vi "Write Frame Data Recorder.vi"(8 "error in (no error)":errorcluster, 9 "Append":bool, 10 "Probe Position":T1, 11 "Frame Grabber Data In in":T5={"Camera Session"="", "Frame"=refnum, "AVI Refnum"=refnum, "Codecs"=[], "Frame number"=0, "Tracking File Refnum"=refnum, "Tick Count"=0, "Probe Object"=refnum, "Playback Probe Data"=[], "Rigid Body"={"Position"={"x (mm)"=0.0, "y (mm)"=0.0, "z (mm)"=0.0}, "Orientation"={"Pitch (rad)"=0.0, "Yaw (rad)"=0.0, "Roll (rad)"=0.0}, "Quaternion"={"qx"=0.0, "qy"=0.0, "qz"=0.0, "qw"=0.0}, "Tracked?"=FALSE}, "Total no frames playback"=0, "Video FPS"=0.0, "Camera connected?"=FALSE, "Scene"=refnum, "Cropped Frame"=refnum, "Tracker FPS"=0.0, "Crop ROI"=[], "Presentation Values"=[], "Elapsed time (ms)"=0, "Camera frames playback"=0, "Refnums"={"Live Refnum"=refnum, "Record Refnum"=refnum, "Playback Refnum"=refnum, "Frame Slider Refnum"=refnum, "Pause Refnum"=refnum, "Home Refnum"=refnum, "Set Crop Refnum"=refnum, "Clear Crop Refnum"=refnum, "stop refnum"=refnum, "Playback Rate Refnum"=refnum, "Presentation Refnum"=refnum, "Crop Time Frame Slider Refnum"=refnum, "Cancel Save Refnum"=refnum, "Reverse Playback Refnum"=refnum, "Recording Settings Refnum"=refnum, "Continuous Playback Refnum"=refnum, "Camera Frame Refnum"=refnum, "Annotation Refnum"=refnum, "Export All Refnum"=refnum, "Export List Refnum"=refnum, "Fill List Refnum"=refnum, "Save Crop Refnum"=refnum, "Skip Forward Refnum"=refnum, "Skip Backward Refnum"=refnum, "Single Annotation Refnum"=refnum, "Load Refnum"=refnum, "Set Start Refnum"=refnum, "Set End Refnum"=refnum, "Add to List Refnum"=refnum, "List of Annotations Refnum"=refnum}, "Dimensions"={"Probe Dimensions"={"Probe Width"=0.0, "Probe Depth"=1.0, "Probe Height"=0.0}, "Room Dimensions"={"Room Width"=0.0, "Room Depth"=0.0, "Room Height"=0.0}}, "Playback Data As Strings"=[], "Cropped Tracking File Refnum"=refnum, "Cropped AVI Refnum"=refnum, "Header"=[], "Total euclidian distance"=0.0, "Annotation File Path"=path "", "Playback File Path"=path "", "Size per frame"=0.0, "Ground Truth File Refnum"=refnum, "Annotation Array"=[], "Annotation TIFFs Folder"=path ""}) -> (0 "error out":errorcluster, 1 "Time elapsed (s)":dbl, 2 "Image":T4, 3 "Frame Grabber Data out":T5={"Camera Session"="", "Frame"=refnum, "AVI Refnum"=refnum, "Codecs"=[], "Frame number"=0, "Tracking File Refnum"=refnum, "Tick Count"=0, "Probe Object"=refnum, "Playback Probe Data"=[], "Rigid Body"={"Position"={"x (mm)"=0.0, "y (mm)"=0.0, "z (mm)"=0.0}, "Orientation"={"Pitch (rad)"=0.0, "Yaw (rad)"=0.0, "Roll (rad)"=0.0}, "Quaternion"={"qx"=0.0, "qy"=0.0, "qz"=0.0, "qw"=0.0}, "Tracked?"=FALSE}, "Total no frames playback"=0, "Video FPS"=0.0, "Camera connected?"=FALSE, "Scene"=refnum, "Cropped Frame"=refnum, "Tracker FPS"=0.0, "Crop ROI"=[], "Presentation Values"=[], "Elapsed time (ms)"=0, "Camera frames playback"=0, "Refnums"={"Live Refnum"=refnum, "Record Refnum"=refnum, "Playback Refnum"=refnum, "Frame Slider Refnum"=refnum, "Pause Refnum"=refnum, "Home Refnum"=refnum, "Set Crop Refnum"=refnum, "Clear Crop Refnum"=refnum, "stop refnum"=refnum, "Playback Rate Refnum"=refnum, "Presentation Refnum"=refnum, "Crop Time Frame Slider Refnum"=refnum, "Cancel Save Refnum"=refnum, "Reverse Playback Refnum"=refnum, "Recording Settings Refnum"=refnum, "Continuous Playback Refnum"=refnum, "Camera Frame Refnum"=refnum, "Annotation Refnum"=refnum, "Export All Refnum"=refnum, "Export List Refnum"=refnum, "Fill List Refnum"=refnum, "Save Crop Refnum"=refnum, "Skip Forward Refnum"=refnum, "Skip Backward Refnum"=refnum, "Single Annotation Refnum"=refnum, "Load Refnum"=refnum, "Set Start Refnum"=refnum, "Set End Refnum"=refnum, "Add to List Refnum"=refnum, "List of Annotations Refnum"=refnum}, "Dimensions"={"Probe Dimensions"={"Probe Width"=0.0, "Probe Depth"=1.0, "Probe Height"=0.0}, "Room Dimensions"={"Room Width"=0.0, "Room Depth"=0.0, "Room Height"=0.0}}, "Playback Data As Strings"=[], "Cropped Tracking File Refnum"=refnum, "Cropped AVI Refnum"=refnum, "Header"=[], "Total euclidian distance"=0.0, "Annotation File Path"=path "", "Playback File Path"=path "", "Size per frame"=0.0, "Ground Truth File Refnum"=refnum, "Annotation Array"=[], "Annotation TIFFs Folder"=path ""}, 4 "File Size (MB)":dbl, 5 "Greater than 2 GB?":bool)   [LabVIEW 2017]
uses:
  Controls/Frame Grabber Data.ctl
  <vilib>/userdefined/High Color/IMAQdx.ctl
  <vilib>/vision/Image Controls.llb/IMAQ Image.ctl
  <vilib>/vision/Avi.llb/IMAQ AVI2 Refnum.ctl
  Controls/Rigid Body Info.ctl
  Controls/Position.ctl
  Controls/Orientation.ctl
  Controls/Refnums.ctl
  Controls/Recording Settings.ctl
  Controls/Operator Settings.ctl
  Controls/Operator.ctl
  Controls/Patient Settings.ctl
  Controls/Dimensions.ctl
  Controls/Room Dimensions.ctl
panel:
  out "Camera frame number":dbl
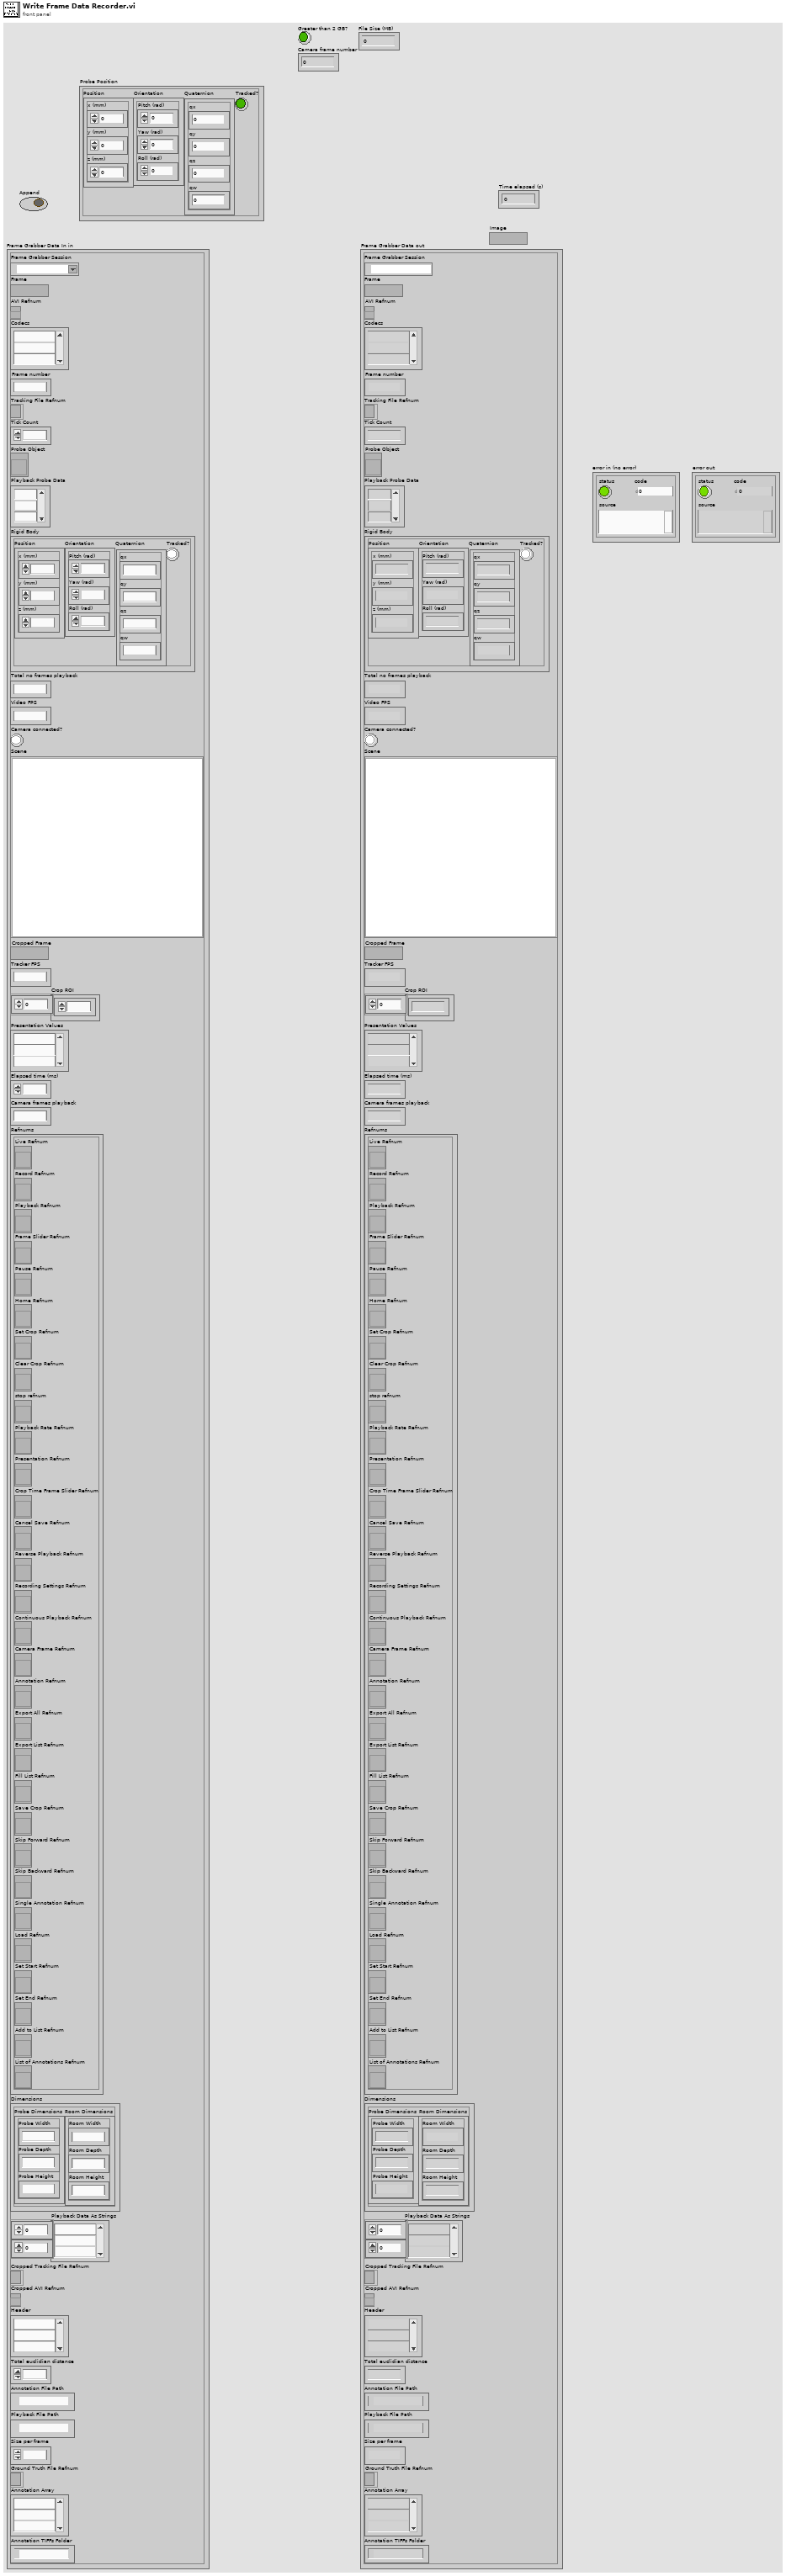
[diagram p1: front panel]
types:
  T1 = typedef "Rigid Body Info.ctl" = cluster{"Position":T2, "Orientation":T3, "Quaternion":cluster{"qx":sgl, "qy":sgl, "qz":sgl, "qw":sgl}, "Tracked?":bool}
  T2 = typedef "Position.ctl" = cluster{"x (mm)":sgl, "y (mm)":sgl, "z (mm)":sgl}
  T3 = typedef "Orientation.ctl" = cluster{"Pitch (rad)":sgl, "Yaw (rad)":sgl, "Roll (rad)":sgl}
  T4 = typedef "IMAQ Image.ctl" = refnum<image>
  T5 = typedef "Frame Grabber Data.ctl" = cluster{"Camera Session":T6, "Frame":T4, "AVI Refnum":T7, "Codecs":string[], "Frame number":u32, "Tracking File Refnum":refnum<file>, "Tick Count":u32, "Probe Object":refnum<vi>, "Playback Probe Data":dbl[][], "Rigid Body":T1, "Total no frames playback":i32, "Video FPS":dbl, "Camera connected?":bool, "Scene":refnum<vi>, "Cropped Frame":T4, "Tracker FPS":dbl, "Crop ROI":i32[], "Presentation Values":string[], "Elapsed time (ms)":u32, "Camera frames playback":u32, "Refnums":T8, "Dimensions":T9, "Playback Data As Strings":string[][], "Cropped Tracking File Refnum":refnum<file>, "Cropped AVI Refnum":T7, "Header":string[], "Total euclidian distance":dbl, "Annotation File Path":path, "Playback File Path":path, "Size per frame":dbl, "Ground Truth File Refnum":refnum<file>, "Annotation Array":string[], "Annotation TIFFs Folder":path}
  T6 = typedef "IMAQdx.ctl" = refnum<k21>
  T7 = typedef "IMAQ AVI2 Refnum.ctl" = refnum<k20>
  T8 = typedef "Refnums.ctl" = cluster{"Live Refnum":refnum<vi>, "Record Refnum":refnum<vi>, "Playback Refnum":refnum<vi>, "Frame Slider Refnum":refnum<vi>, "Pause Refnum":refnum<vi>, "Home Refnum":refnum<vi>, "Set Crop Refnum":refnum<vi>, "Clear Crop Refnum":refnum<vi>, "stop refnum":refnum<vi>, "Playback Rate Refnum":refnum<vi>, "Presentation Refnum":refnum<vi>, "Crop Time Frame Slider Refnum":refnum<vi>, "Cancel Save Refnum":refnum<vi>, "Reverse Playback Refnum":refnum<vi>, "Recording Settings Refnum":refnum<vi>, "Continuous Playback Refnum":refnum<vi>, "Camera Frame Refnum":refnum<vi>, "Annotation Refnum":refnum<vi>, "Export All Refnum":refnum<vi>, "Export List Refnum":refnum<vi>, "Fill List Refnum":refnum<vi>, "Save Crop Refnum":refnum<vi>, "Skip Forward Refnum":refnum<vi>, "Skip Backward Refnum":refnum<vi>, "Single Annotation Refnum":refnum<vi>, "Load Refnum":refnum<vi>, "Set Start Refnum":refnum<vi>, "Set End Refnum":refnum<vi>, "Add to List Refnum":refnum<vi>, "List of Annotations Refnum":refnum<vi>}
  T9 = typedef "Dimensions.ctl" = cluster{"Probe Dimensions":cluster{"Probe Width":sgl, "Probe Depth":sgl, "Probe Height":sgl}, "Room Dimensions":T10}
  T10 = typedef "Room Dimensions.ctl" = cluster{"Room Width":dbl, "Room Depth":dbl, "Room Height":dbl}
  T11 = typedef "Recording Settings.ctl" = cluster{"Folder to Save Recordings":path, "Video FPS":u32, "Codec":u16, "Tracker FPS":u32, "Operator ID":T12, "Patient ID/Gestation":T14}
  T12 = typedef "Operator Settings.ctl" = cluster{"Operator ID":u32, "Expertise":T13}
  T13 = typedef "Operator.ctl" = u16
  T14 = typedef "Patient Settings.ctl" = cluster{"ID":u32, "Gestation":string}
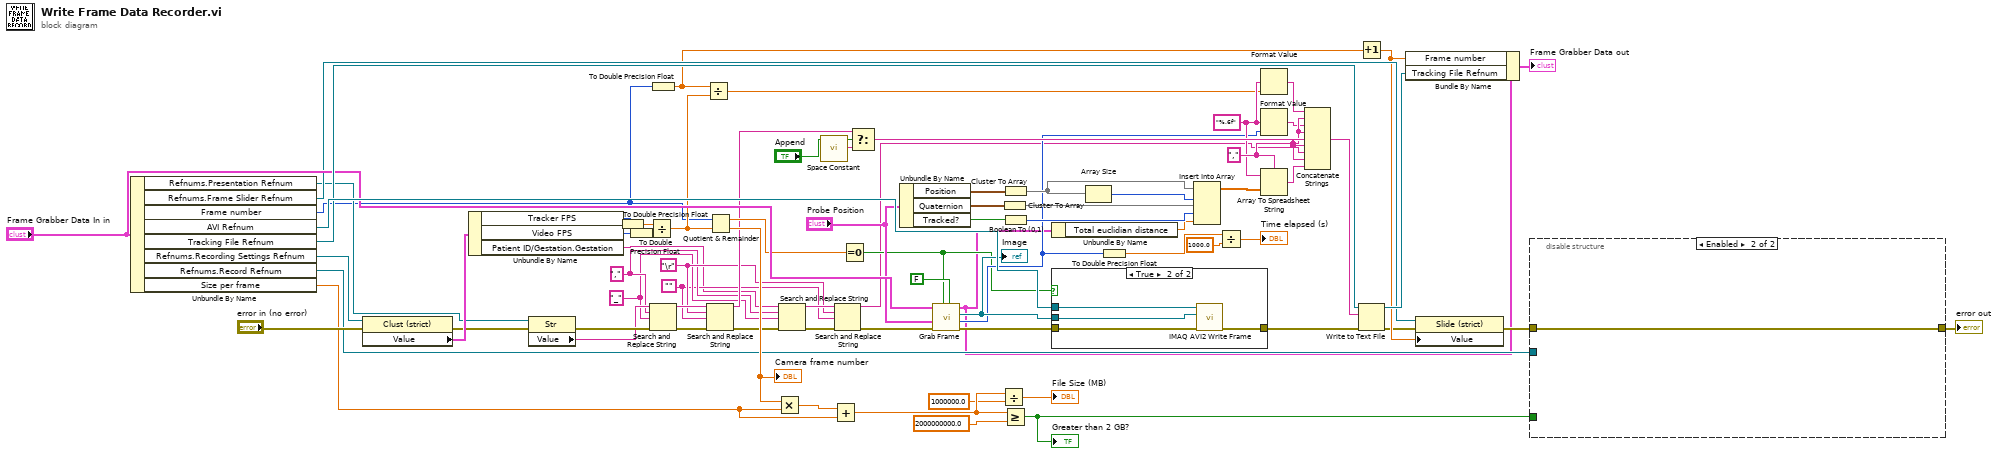
[diagram p0: block diagram]
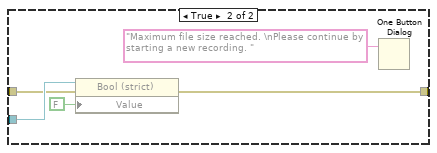
[diagram p3: hidden frame]
diagram:
  w9 = ""
  w12 = "\r"
  w10 = "_" ("replace string (\"\")")
  w11 = "," ("search string")
  w46 = "," ("delimiter (Tab)")
  w45 = "%.6f" ("format string")
  n1 = Unbundle By Name("Frame Grabber Data In in") -> ("Refnums.Presentation Refnum"=w36:refnum<vi>, "Refnums.Frame Slider Refnum"=w58:refnum<vi>, "Frame number"=w32:u32, "AVI Refnum"=w76:T7, "Tracking File Refnum"=w75:refnum<file>, "Refnums.Recording Settings Refnum"=w39:refnum<vi>, "Refnums.Record Refnum"=w23:refnum<vi>, "Size per frame"=w4:dbl)
  n2 = property class="Clust (strict)"(reference=w39, error in="error in (no error)") -> (error out=w35:errorcluster, "Value"=w38:T11)  [unwired: 1 out]
  n3 = Unbundle By Name(w38) -> ("Tracker FPS"=w54:u32, "Video FPS"=w51:u32, "Patient ID/Gestation.Gestation"=w3:string)
  n4 = property class="Str"(reference=w36, error in=w35) -> (error out=w22:errorcluster, "Value"=w21:string)  [unwired: 1 out]
  n5 = To Double Precision Float(number=w54) -> (double precision float=w2:dbl)
  n6 = To Double Precision Float(number=w51) -> (double precision float=w1:dbl)
  n7 = Divide(x=w2, y=w1) -> (x/y=w47:dbl)
  n8 = Search and Replace String(input string=w21, search string=w11, replace string=w10, error in=w22) -> (result string=w18:string, error out=w20:errorcluster)  [unwired: 4 in, 2 out]
  n9 = To Double Precision Float(number=w32) -> (double precision float=w34:dbl)
  n10 = Divide(x=w34, y=w47) -> (x/y=w33:dbl)
  n11 = Search and Replace String(input string=w18, search string=w12, replace string=w9, error in=w20) -> (result string=w17:string, error out=w19:errorcluster)  [unwired: 4 in, 2 out]
  n12 = Quotient & Remainder(x=w32, y=w47) -> (x-y*floor(x/y)=w52:dbl, floor(x/y)=w30:dbl)
  "Camera frame number" <- w30
  n13 = Multiply(x=w30, y=w4) -> (x*y=w29:dbl)
  n14 = Search and Replace String(input string=w3, search string=w11, replace string=w10, error in=w19) -> (result string=w15:string, error out=w16:errorcluster)  [unwired: 4 in, 2 out]
  n15 = call <vilib>:"Space Constant.vi"() -> ("String"=w55:string)
  n16 = Add(x=w29, y=w4) -> (x+y=w27:dbl)
  n17 = Search and Replace String(input string=w15, search string=w12, replace string=w9, error in=w16) -> (result string=w14:string, error out=w13:errorcluster)  [unwired: 4 in, 2 out]
  n18 = Equal To 0?(x=w52) -> (x = 0?=w31:bool)
  n19 = Select(t=w17, s="Append", f=w55) -> (s? t:f=w48:string)
  n20 = Unbundle By Name("Probe Position") -> ("Position"=w69:T2, "Quaternion"=w73:cluster{"qx":sgl, "qy":sgl, "qz":sgl, "qw":sgl}, "Tracked?"=w60:bool)
  n21 = call "Grab Frame.vi"("Live?"=FALSE, "Grab frame?"=w31, "error in (no error)"=w13, "Rigid Body"="Probe Position", "Frame Grabber Data in"="Frame Grabber Data In in") -> ("error out"=w64:errorcluster, "Elapsed time (ms)"=w43:u32, "Frame"=w65:T4, "Frame Grabber Data out"=w8:T5)  [unwired: 3 in]
  "Image" <- w65
  n22 = Divide(x=w27, y=1000000.0) -> (x/y=→"File Size (MB)":dbl)
  n23 = Cluster To Array(cluster=w73) -> (array=w70:sgl[])
  n24 = Cluster To Array(cluster=w69) -> (array=w71:sgl[])
  n25 = Boolean To (0,1)(Boolean=w60) -> (0, 1=w59:i16)
  n26 = Greater Or Equal?(x=w27, y=2000000000.0) -> (x >= y?=w26:bool)
  "Greater than 2 GB?" <- w26
  n27 = Unbundle By Name(w8) -> ("Total euclidian distance"=w7:dbl)
  n28 = case shown="True" w31 {
    tunnel: [w78 w82] -> w77
    tunnel: w76 -> [_ w81]
    tunnel: w65 -> [_ w80]
    tunnel: w64 -> [w78 w79]
    frame False {
    }
    frame True {
      n29 = call "IMAQ AVI2 Write Frame"("error in (no error)"=w79, "Image"=w80, "AVI Refnum"=w81) -> ("error out"=w82:errorcluster)  [unwired: 6 in, 2 out]
    }
  }
  n30 = Array Size(array=w71) -> (size(s)=w72:i32)
  n31 = To Double Precision Float(number=w43) -> (double precision float=w41:dbl)
  n32 = Insert Into Array(array=w71, index=w72, new element #1=w70, new element #2=w59, new element #3=w7) -> (w74:sgl[])
  n33 = Divide(x=w41, y=1000.0) -> (x/y=→"Time elapsed (s)":dbl)
  n34 = Format Value(format string=w45, value (0)=w33) -> (output string=w49:string)  [unwired: 1 in]
  n35 = Format Value(format string=w45, value (0)=w43) -> (output string=w44:string)  [unwired: 1 in]
  n36 = Array To Spreadsheet String(delimiter (Tab)=w46, array=w74, 3:w45) -> (spreadsheet string=w68:string)
  n37 = Concatenate Strings(w49, w46, w44, w46, w48, w46, w14, w46, w68) -> (w67:string)
  n38 = Increment(x=w34) -> (x+1=w57:dbl)
  n39 = Write to Text File(file (use dialog)=w75, text=w67, error in=w77) -> (refnum out=w66:refnum<file>, error out=w56:errorcluster)  [unwired: 1 in, 1 out]
  n40 = Bundle By Name(cluster=w8, "Frame number"=w57, "Tracking File Refnum"=w66) -> (→"Frame Grabber Data out":T5)
  n41 = property class="Slide (strict)"(reference=w58, error in=w56, "Value"=w57) -> (error out=w25:errorcluster)  [unwired: 1 out]
  n42 = disable-structure shown="Enabled" {
    disable-tunnel: w26 -> [w86 _]
    disable-tunnel: w25 -> [w85 w93]
    disable-tunnel: [w84 w93] -> w24
    disable-tunnel: w23 -> [w83 _]
    frame Disabled {
      n43 = case shown="False" w86 {
        tunnel: w85 -> [w87 w90]
        tunnel: [w87 w89] -> w84
        tunnel: w83 -> [_ w91]
        frame False {
        }
        frame True {
          n44 = property class="Bool (strict)"(reference=w91, error in=w90, "Value"=FALSE) -> (error out=w89:errorcluster)  [unwired: 1 out]
          n45 = One Button Dialog(message="Maximum file size reached. \nPlease continue by starting a new recording. ") -> ()  [unwired: 1 in, 1 out]
        }
      }
    }
    frame Enabled {
    }
  }
  "error out" <- w24
